vi "Simulate Serial Outpot Random.vi"() -> ()   [LabVIEW 2009]
panel:
  in  "Serial Port":refnum<visa-resource-name>="COM1"
  in  "Seconds to Wait":dbl=10.0 format="%1_4g"
  in  "stop":bool
  in  "FANS":bool
  in  "COMP":bool
  in  "LE":bool
  in  "UE":bool
  out "output":string
  in  "Power On":bool=TRUE
  out "error out":errorcluster
  out "time string":string
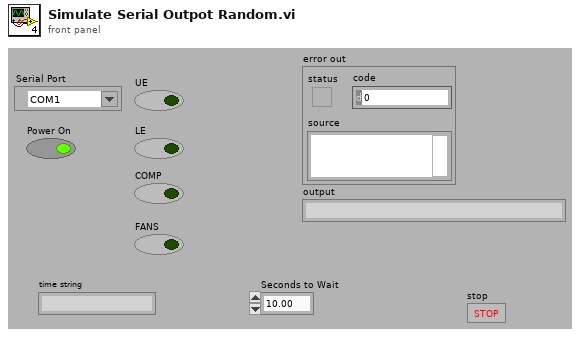
[diagram p1: front panel]
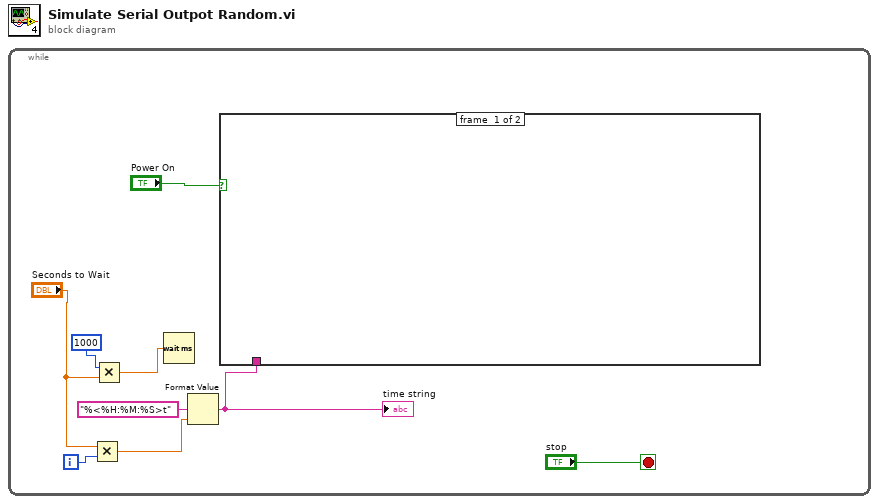
[diagram p0: block diagram]
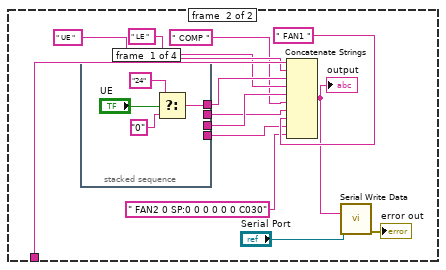
[diagram p2: hidden frame]
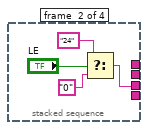
[diagram p3: hidden frame]
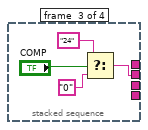
[diagram p4: hidden frame]
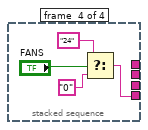
[diagram p5: hidden frame]
diagram:
  n1 = while {
    i -> [w8]
    stop <- "stop" stop-if-true
    n2 = Multiply(x="Seconds to Wait", y=w8) -> (x*y=w6:dbl)
    n3 = Multiply(x=u32 1000 ("milliseconds to wait"), y="Seconds to Wait") -> (x*y=w5:dbl)
    n4 = Wait (ms)(milliseconds to wait=w5) -> ()  [unwired: 1 out]
    n5 = Format Value(format string="%<%H:%M:%S>t", value (0)=w6) -> (output string=w3:string)  [unwired: 1 in]
    "time string" <- w3
    n6 = case shown="True" "Power On" {
      tunnel: w3 -> [_ w21]
      frame #0 {
      }
      frame #1 {
        n7 = stacked-sequence {
          tunnel: [w24 _ _ _] -> w19
          tunnel: [_ w27 _ _] -> w18
          tunnel: [_ _ w31 _] -> w15
          tunnel: [_ _ _ w35] -> w13
          frame #0 {
            n8 = Select(t="24" ("trimmed string"), s="UE", f="0" ("trimmed string")) -> (s? t:f=w24:string)
          }
          frame #1 {
            n9 = Select(t="24" ("trimmed string"), s="LE", f="0" ("trimmed string")) -> (s? t:f=w27:string)
          }
          frame #2 {
            n10 = Select(t="24" ("trimmed string"), s="COMP", f="0" ("trimmed string")) -> (s? t:f=w31:string)
          }
          frame #3 {
            n11 = Select(t="24" ("trimmed string"), s="FANS", f="0" ("trimmed string")) -> (s? t:f=w35:string)
          }
        }
        n12 = Concatenate Strings(w21, " UE " ("trimmed string"), w19, " LE " ("trimmed string"), w18, " COMP " ("trimmed string"), w15, " FAN1 " ("trimmed string"), w13, " FAN2 0 SP:0 0 0 0 0 0 C030" ("trimmed string")) -> (w11:string)
        "output" <- w11
        n13 = call "Serial Write Data.vi"("VISA resource name"="Serial Port", "trimmed string"=w11) -> ("error out"=→"error out":errorcluster)  [unwired: 13 in]
      }
    }
  }
